vi "PRIMA ARRAY.vi"() -> ()   [LabVIEW 2017]
panel:
  out "Array":i32[](array[numeric])
  out "Numeric":dbl
  in  "Batas Angka":u64 min=2
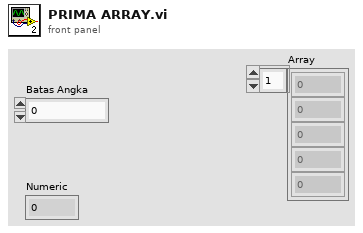
[diagram p1: front panel]
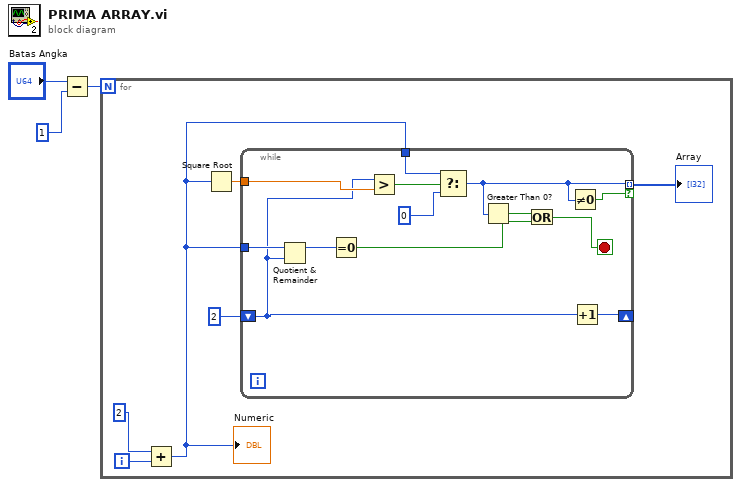
[diagram p0: block diagram]
diagram:
  n1 = Subtract(x="Batas Angka", y=1) -> (x-y=w3:u64)
  n2 = for {
    N: w3 -> [_]
    i -> [w5]
    n3 = Add(x=2, y=w5) -> (x+y=w6:i32)
    "Numeric" <- w6
    n4 = Square Root(x=w6) -> (sqrt(x)=w9:dbl)
    n5 = while {
      tunnel: w6 -> [w22]
      tunnel: w9 -> [w20]
      shift-right: [w21] -> _
      shift-left: u32 2 -> [w17]
      tunnel: w6 -> [w13]
      tunnel: [w10] -> w4 mode=indexing if=w11
      stop <- w14 stop-if-true
      n6 = Quotient & Remainder(x=w22, y=w17) -> (x-y*floor(x/y)=w18:u32)  [unwired: 1 out]
      n7 = Equal To 0?(x=w18) -> (x = 0?=w15:bool)
      n8 = Greater?(x=w17, y=w20) -> (0:w19:bool)
      n9 = Select(t=w13, s=w19, f=0) -> (s? t:f=w10:i32)
      n10 = Greater Than 0?(x=w10) -> (x > 0?=w16:bool)
      n11 = Or(x=w16, y=w15) -> (x .or. y?=w14:bool)
      n12 = Not Equal To 0?(x=w10) -> (x != 0?=w11:bool)
      n13 = Increment(x=w17) -> (x+1=w21:u32)
    }
    "Array" <- w4
  }
